vi "Periodic Tasks.vi"(0 "error in":errorcluster) -> ()   [LabVIEW 2020]
doc: "All TeleOperated, Autonomous, and Test controller logic are located here. Sensor reads and actuator commands are run inside of parallel loops. Most FRC 4265 code should be placed here."
uses:
  b6b65418-eac7-4813-9cbe-065ecdd83a5a.vi
  sensors.vi
  dsdata.vi
  dscommands.vi
  outputs.vi
  autoninfo.vi
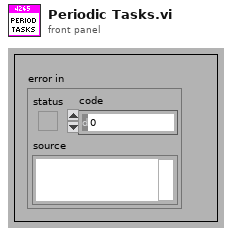
[diagram p1: front panel]
types:
  T1 = typedef "WPI_DriverStationRobotMode2.ctl" = enum16{"Autonomous Disabled", "Autonomous Enabled", "Teleop Disabled", "Teleop Enabled", "Disconnected", "Finish", "Test Disabled", "Test Enabled", "Emergency Stopped"}
  T2 = cluster{"Auto Error Out":errorcluster, "Drive Advance":bool, "Drive Step":i32, "Manipulator Step":i32, "Manipulator Advance":bool}
  T3 = cluster{"Auto Error":errorcluster, "Drive Advance":bool, "Drive Step":i32, "Manipulator Step":i32, "Manipulator Advance":bool}
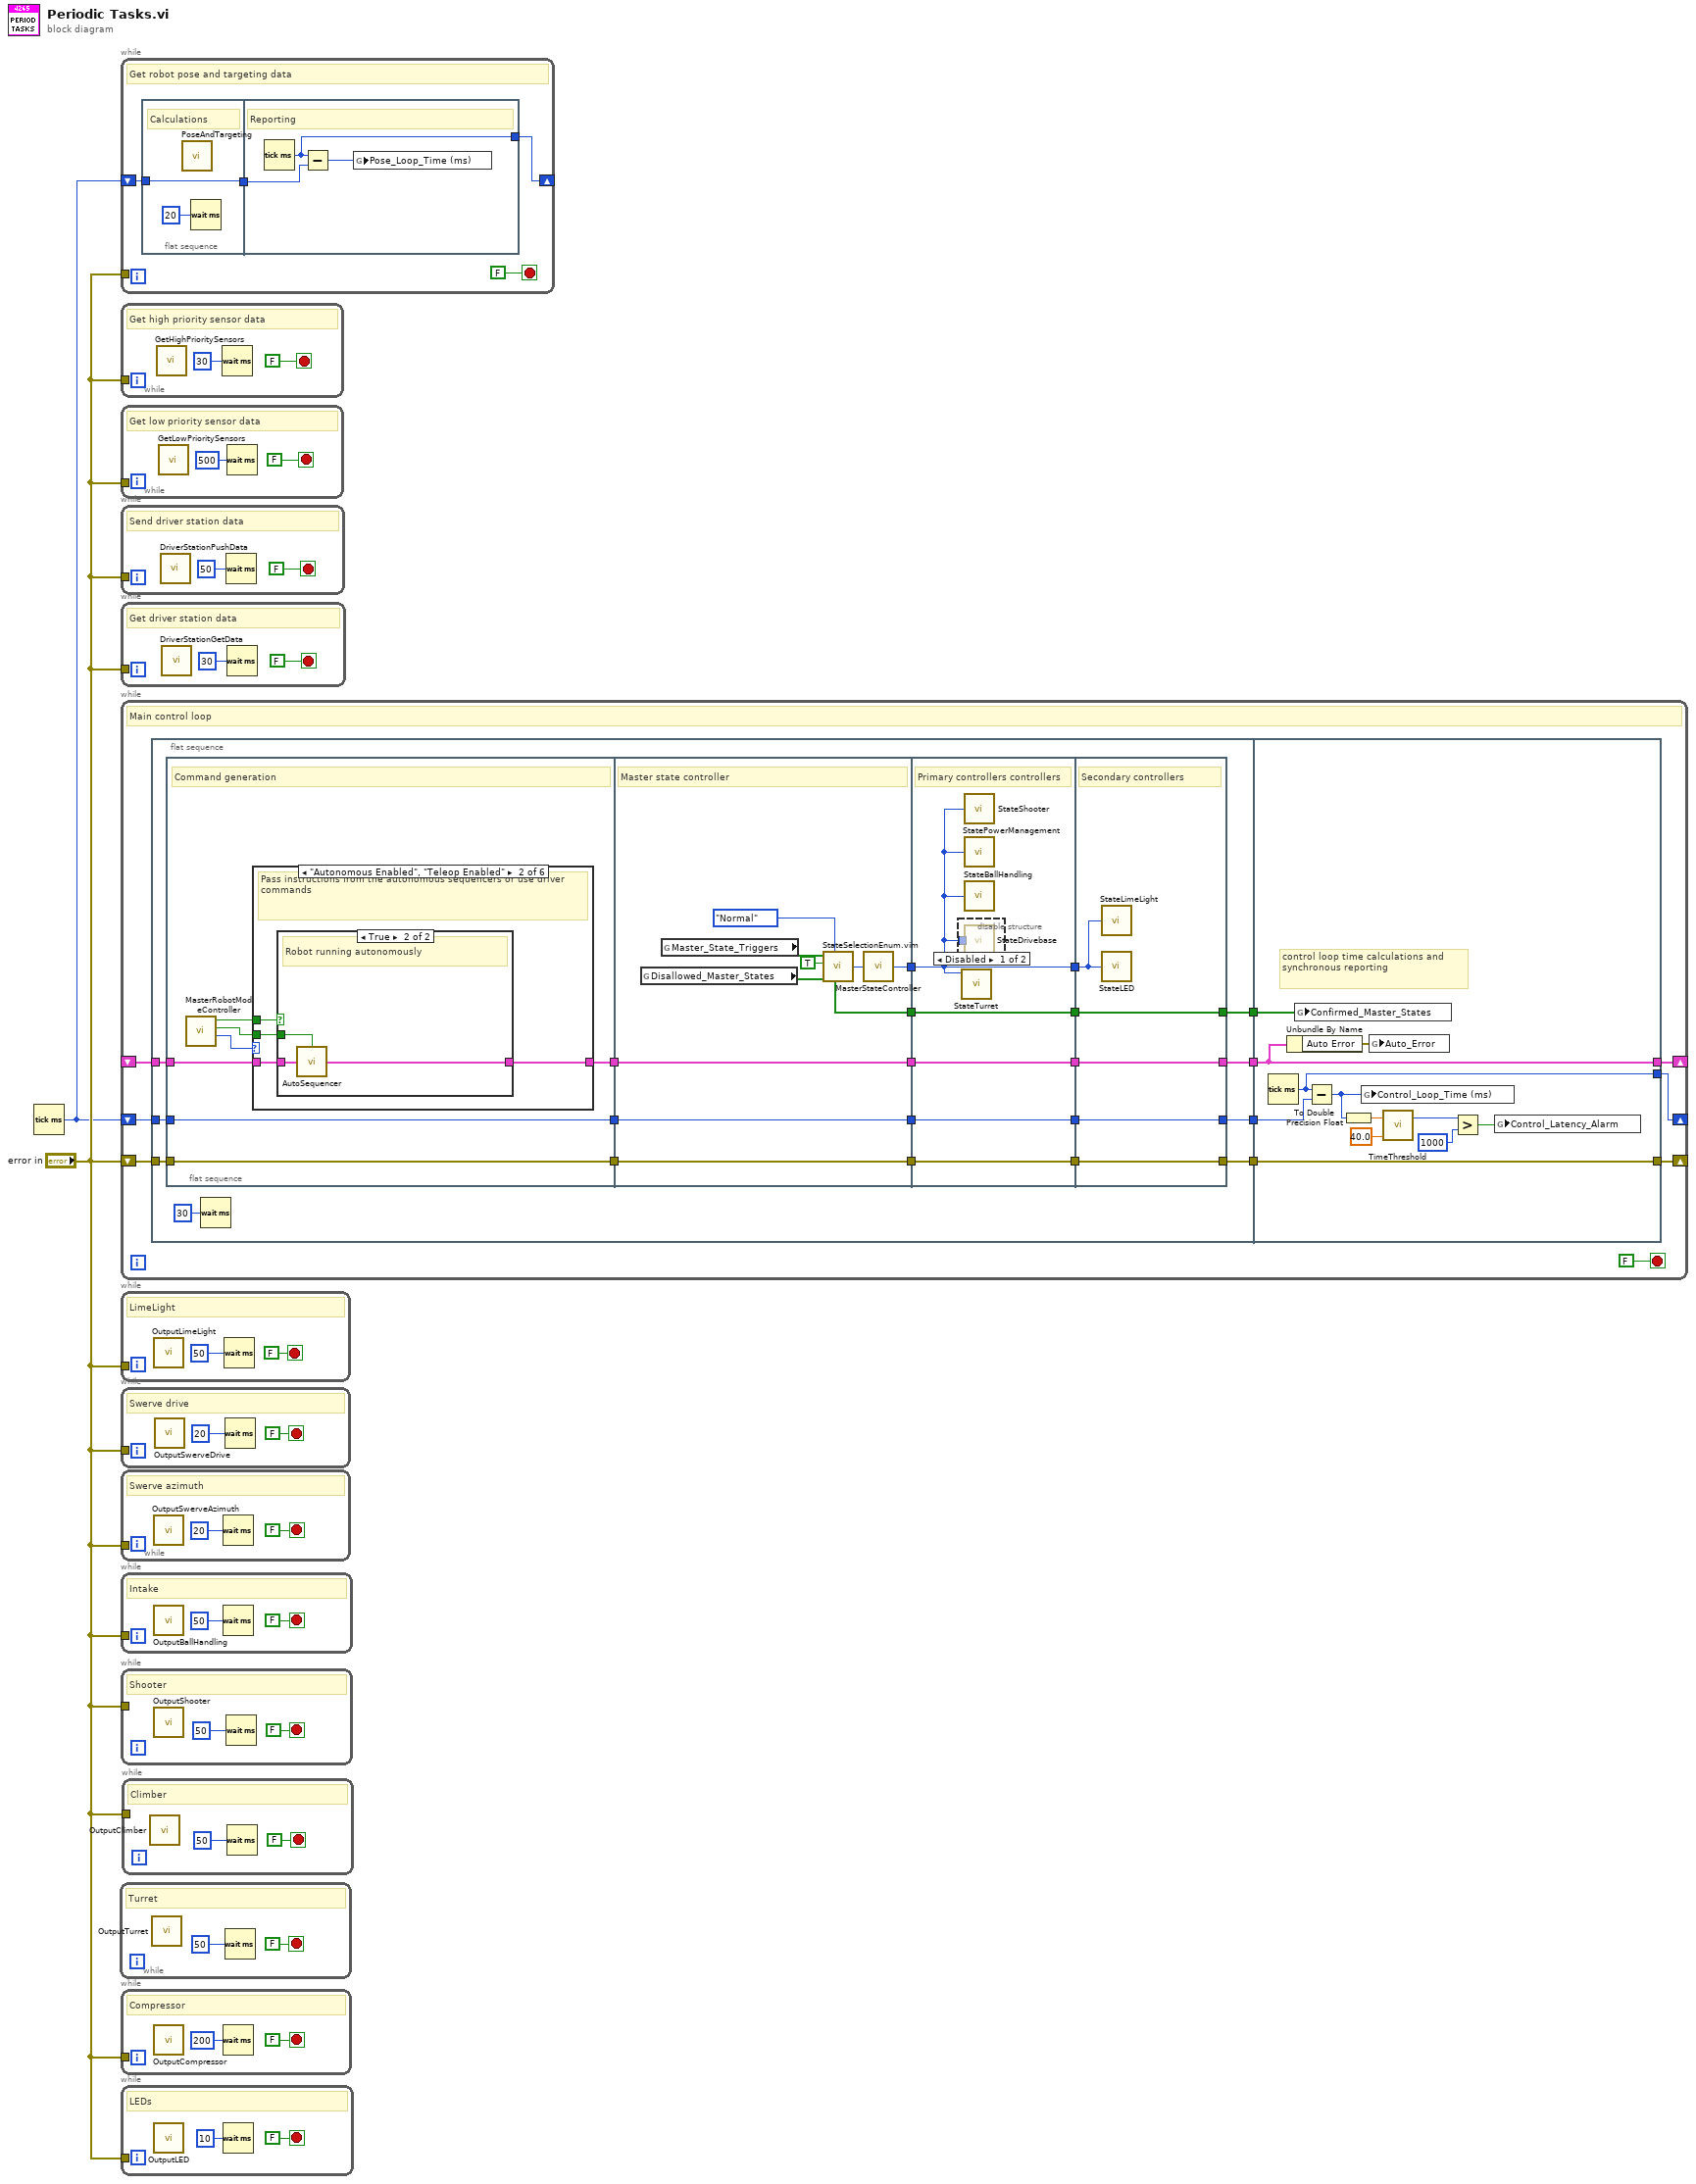
[diagram p0: block diagram]
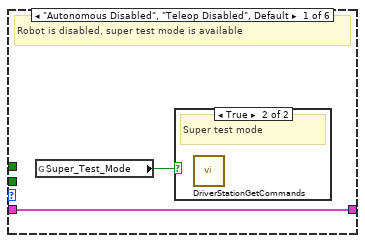
[diagram p2: hidden frame]
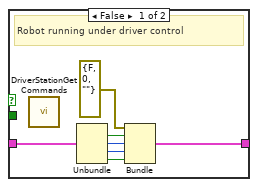
[diagram p4: hidden frame]
diagram:
  n1 = Tick Count (ms)() -> (millisecond timer value=w1:u32)
  n2 = while {
    stop <- FALSE stop-if-true
    # "Turret"
    n3 = call "OutputTurret.vi"() -> ()  [unwired: 1 in]
    n4 = Wait (ms)(milliseconds to wait=u32 50) -> ()  [unwired: 1 out]
  }
  n5 = while {
    tunnel: "error in" -> [_]
    shift-right: [w7] -> _
    shift-left: w1 -> [w6]
    stop <- FALSE stop-if-true
    # "Get robot pose and targeting data"
    n6 = flat-sequence {
      tunnel: w6 -> [w10]
      tunnel: [w10] -> w5
      tunnel: [w12] -> w7
      tunnel: w5 -> [w11]
      frame #0 {
        # "Calculations"
        n7 = call "PoseAndTargeting.vi"() -> ()  [unwired: 1 in]
        n8 = Wait (ms)(milliseconds to wait=u32 20) -> ()  [unwired: 1 out]
      }
      frame #1 {
        # "Reporting"
        n9 = Tick Count (ms)() -> (millisecond timer value=w12:u32)
        n10 = Subtract(x=w12, y=w11) -> (x-y=w13:u32)
        n11 = global write "sensors.vi" "Pose_Loop_Time (ms)"(w13) -> ()
      }
    }
  }
  n12 = while {
    tunnel: "error in" -> [_]
    stop <- FALSE stop-if-true
    # "Get high priority sensor data"
    n13 = call "GetHighPrioritySensors.vi"() -> ()  [unwired: 1 in]
    n14 = Wait (ms)(milliseconds to wait=u32 30) -> ()  [unwired: 1 out]
  }
  n15 = while {
    tunnel: "error in" -> [_]
    stop <- FALSE stop-if-true
    # "Get low priority sensor data"
    n16 = call "GetLowPrioritySensors.vi"() -> ()  [unwired: 1 in]
    n17 = Wait (ms)(milliseconds to wait=u32 500) -> ()  [unwired: 1 out]
  }
  n18 = while {
    tunnel: "error in" -> [_]
    stop <- FALSE stop-if-true
    # "Send driver station data"
    n19 = call "DriverStationPushData.vi"() -> ()  [unwired: 1 in]
    n20 = Wait (ms)(milliseconds to wait=u32 50) -> ()  [unwired: 1 out]
  }
  n21 = while {
    tunnel: "error in" -> [_]
    stop <- FALSE stop-if-true
    # "Get driver station data"
    n22 = call "DriverStationGetData.vi"() -> ()  [unwired: 1 in]
    n23 = Wait (ms)(milliseconds to wait=u32 30) -> ()  [unwired: 1 out]
  }
  n24 = while {
    shift-right: [w26] -> _
    shift-left: w1 -> [w27]
    shift-right: [w31] -> _
    shift-left: _ -> [w30]
    shift-right: [w28] -> _
    shift-left: "error in" -> [w29]
    stop <- FALSE stop-if-true
    # "Main control loop"
    n25 = flat-sequence {
      tunnel: w30 -> [w42]
      tunnel: w29 -> [w41]
      tunnel: w27 -> [w39]
      tunnel: [w43] -> w25
      tunnel: [w40] -> w24
      tunnel: [w37] -> w23
      tunnel: [w33] -> w22
      tunnel: [w105] -> w26
      tunnel: [w113] -> w28
      tunnel: [w103] -> w31
      tunnel: w25 -> [w103]
      tunnel: w24 -> [w113]
      tunnel: w23 -> [w106]
      tunnel: w22 -> [w104]
      frame #0 {
        n26 = flat-sequence {
          tunnel: [w60] -> w53
          tunnel: w42 -> [w59]
          tunnel: [w55] -> w52
          tunnel: w41 -> [w55]
          tunnel: [w54] -> w51
          tunnel: w39 -> [w54]
          tunnel: [w90] -> w50
          tunnel: [w89] -> w49
          tunnel: w53 -> [w89]
          tunnel: w52 -> [w88]
          tunnel: [w88] -> w48
          tunnel: w51 -> [w87]
          tunnel: [w87] -> w47
          tunnel: [w82] -> w34
          tunnel: w50 -> [w91]
          tunnel: [w95] -> w46
          tunnel: w49 -> [w95]
          tunnel: [w94] -> w45
          tunnel: w48 -> [w94]
          tunnel: [w93] -> w44
          tunnel: w47 -> [w93]
          tunnel: [w91] -> w36
          tunnel: [w92] -> w35
          tunnel: w34 -> [w92]
          tunnel: [w101] -> w43
          tunnel: w46 -> [w101]
          tunnel: [w100] -> w40
          tunnel: w45 -> [w100]
          tunnel: w44 -> [w99]
          tunnel: [w99] -> w37
          tunnel: w36 -> [w98]
          tunnel: [w97] -> w33
          tunnel: w35 -> [w97]
          frame #0 {
            # "Command generation"
            n27 = call "MasterRobotModeController.vi"() -> ("FMS Robot Mode"=w58:T1, "Auto Reset"=w57:bool, "Robot is Autonomous"=w56:bool)  [unwired: 5 in]
            n28 = case shown="\"Autonomous Enabled\", \"Teleop Enabled\"" w58 {
              tunnel: w57 -> [_ w64 _ _ _ _]
              tunnel: [w61 w66 w77 w78 w79 w80] -> w60
              tunnel: w59 -> [w61 w65 w77 w78 w79 w80]
              tunnel: w56 -> [_ w63 _ _ _ _]
              frame "Autonomous Disabled", "Teleop Disabled", Default {
                # "Robot is disabled, super test mode is available"
                n29 = global read "dsdata.vi" "Super_Test_Mode"() -> (w62:bool)
                n30 = case shown="True" w62 {
                  frame False {
                    # "Fully disabled"
                  }
                  frame True {
                    # "Super test mode"
                    n31 = call "DriverStationGetCommands.vi"() -> ()  [unwired: 12 in]
                  }
                }
              }
              frame "Autonomous Enabled", "Teleop Enabled" {
                # "Pass instructions from the autonomous sequencers or use driver commands"
                n32 = case shown="True" w63 {
                  tunnel: w64 -> [_ w76]
                  tunnel: [w72 w75] -> w66
                  tunnel: w65 -> [w73 w74]
                  frame False {
                    # "Robot running under driver control"
                    n33 = call "DriverStationGetCommands.vi"() -> ()  [unwired: 12 in]
                    n34 = Unbundle(w73) -> ("Drive Advance"=w68:bool, "Drive Step"=w69:i32, "Manipulator Step"=w70:i32, "Manipulator Advance"=w71:bool)  [unwired: 1 out]
                    n35 = Bundle("Auto Error Out"=errorcluster {"status"=FALSE, "code"=0, "source"=""}, "Drive Advance"=w68, "Drive Step"=w69, "Manipulator Step"=w70, "Manipulator Advance"=w71) -> (w72:T2)  [unwired: 1 in]
                  }
                  frame True {
                    # "Robot running autonomously"
                    n36 = call "AutoSequencer.vi"("Reinit Sequencer"=w76, "Auto Cluster In"=w74) -> ("Auto Cluster Out"=w75:T3)  [unwired: 13 in]
                  }
                }
              }
              frame "Finish" {
                # "Clean up operations are in the Finish.vi in RobotMain.vi"
              }
              frame "Test Disabled", "Test Enabled" {
                # "Use TestActuatorInterlock.vi for implimenting test code"
              }
              frame "Disconnected" {
                # "Communications have failed"
              }
              frame "Emergency Stopped" {
                # "Robot has been emergency stopped"
              }
            }
          }
          frame #1 {
            # "Master state controller"
            n37 = global read "outputs.vi" "Disallowed_Master_States"() -> (w85:bool[])
            n38 = global read "dscommands.vi" "Master_State_Triggers"() -> (w86:bool[])
            n39 = call "StateSelectionEnum.vim"("Enum Def"=enum16{"Normal", "Climb"}."Normal", "Disallowed States"=w85, "Enable Edge Trigger"=TRUE, "State Triggers"=w86) -> ("Selected State"=w83:enum16{"Normal", "Climb"}, "Confirmed States"=w82:bool[])  [unwired: 1 in]
            n40 = call "MasterStateController.vi"("Master State In"=w83) -> ("Master State Out"=w90:enum16{"Normal", "Climb"})
          }
          frame #2 {
            # "Primary controllers controllers"
            n41 = disable-structure shown="Disabled" {
              disable-tunnel: w91 -> [w96 _]
              frame Disabled {
                n42 = call "StateDrivebase.vi"("Master State"=w96) -> ()
              }
              frame Enabled {
              }
            }
            n43 = call "StateTurret.vi"("Master State"=w91) -> ()  [unwired: 11 in]
            n44 = call "StateShooter.vi"("Master State"=w91) -> ()
            n45 = call "StatePowerManagement.vi"("Master State"=w91) -> ()
            n46 = call "StateBallHandling.vi"("Master State"=w91) -> ()
          }
          frame #3 {
            # "Secondary controllers"
            n47 = call "StateLimeLight.vi"("Master State"=w98) -> ()
            n48 = call "StateLED.vi"("Master State"=w98) -> ()
          }
        }
        n49 = Wait (ms)(milliseconds to wait=u32 30) -> ()  [unwired: 1 out]
      }
      frame #1 {
        # "control loop time calculations and synchronous reporting"
        n50 = Tick Count (ms)() -> (millisecond timer value=w105:u32)
        n51 = Unbundle By Name(w103) -> ("Auto Error"=w102:errorcluster)
        n52 = global write "outputs.vi" "Confirmed_Master_States"(w104) -> ()
        n53 = Subtract(x=w105, y=w106) -> (x-y=w112:u32)
        n54 = To Double Precision Float(number=w112) -> (double precision float=w111:dbl)
        n55 = global write "sensors.vi" "Control_Loop_Time (ms)"(w112) -> ()
        n56 = global write "autoninfo.vi" "Auto_Error"(w102) -> ()
        n57 = call "TimeThreshold.vi"("Threshold"=40.0, "Current Value"=w111) -> ("Time Above Threshold (ms)"=w110:u32)  [unwired: 1 out]
        n58 = Greater?(x=w110, y=u32 1000) -> (0:w109:bool)
        n59 = global write "sensors.vi" "Control_Latency_Alarm"(w109) -> ()
      }
    }
  }
  n60 = while {
    tunnel: "error in" -> [_]
    stop <- FALSE stop-if-true
    # "LimeLight"
    n61 = call "OutputLimeLight.vi"() -> ()  [unwired: 1 in]
    n62 = Wait (ms)(milliseconds to wait=u32 50) -> ()  [unwired: 1 out]
  }
  n63 = while {
    tunnel: "error in" -> [_]
    stop <- FALSE stop-if-true
    # "Swerve drive"
    n64 = call "OutputSwerveDrive.vi"() -> ()  [unwired: 1 in]
    n65 = Wait (ms)(milliseconds to wait=u32 20) -> ()  [unwired: 1 out]
  }
  n66 = while {
    tunnel: "error in" -> [_]
    stop <- FALSE stop-if-true
    # "Swerve azimuth"
    n67 = call "OutputSwerveAzimuth.vi"() -> ()  [unwired: 1 in]
    n68 = Wait (ms)(milliseconds to wait=u32 20) -> ()  [unwired: 1 out]
  }
  n69 = while {
    tunnel: "error in" -> [_]
    stop <- FALSE stop-if-true
    # "Intake"
    n70 = call "OutputBallHandling.vi"() -> ()  [unwired: 1 in]
    n71 = Wait (ms)(milliseconds to wait=u32 50) -> ()  [unwired: 1 out]
  }
  n72 = while {
    tunnel: "error in" -> [_]
    stop <- FALSE stop-if-true
    # "Shooter"
    n73 = call "OutputShooter.vi"() -> ()  [unwired: 1 in]
    n74 = Wait (ms)(milliseconds to wait=u32 50) -> ()  [unwired: 1 out]
  }
  n75 = while {
    tunnel: "error in" -> [_]
    stop <- FALSE stop-if-true
    # "Compressor"
    n76 = call "OutputCompressor.vi"() -> ()  [unwired: 1 in]
    n77 = Wait (ms)(milliseconds to wait=u32 200) -> ()  [unwired: 1 out]
  }
  n78 = while {
    tunnel: "error in" -> [_]
    stop <- FALSE stop-if-true
    # "LEDs"
    n79 = call "OutputLED.vi"() -> ()  [unwired: 1 in]
    n80 = Wait (ms)(milliseconds to wait=u32 10) -> ()  [unwired: 1 out]
  }
  n81 = while {
    tunnel: "error in" -> [_]
    stop <- FALSE stop-if-true
    # "Climber"
    n82 = call "OutputClimber.vi"() -> ()  [unwired: 1 in]
    n83 = Wait (ms)(milliseconds to wait=u32 50) -> ()  [unwired: 1 out]
  }
